vi "VR_WR.vi"(6 "Ydrp":dbl[](array[numeric]), 7 "Phirp":dbl[](array[numeric]), 9 "Xdrp":dbl[](array[numeric]), 10 "Phir":dbl[](array[numeric])) -> ()   [LabVIEW 2011]
uses:
  <vilib>/Analysis/Matrix/Datatypes/RealMatrix.ctl
  <vilib>/Analysis/Matrix/NI_Matrix.lvlib
panel:
  out "Real Matrix":T1
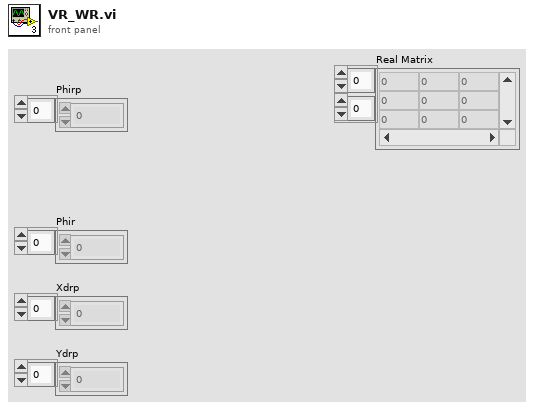
[diagram p1: front panel]
types:
  T1 = typedef "NI_Matrix.lvlib/RealMatrix.ctl" = dbl[][]
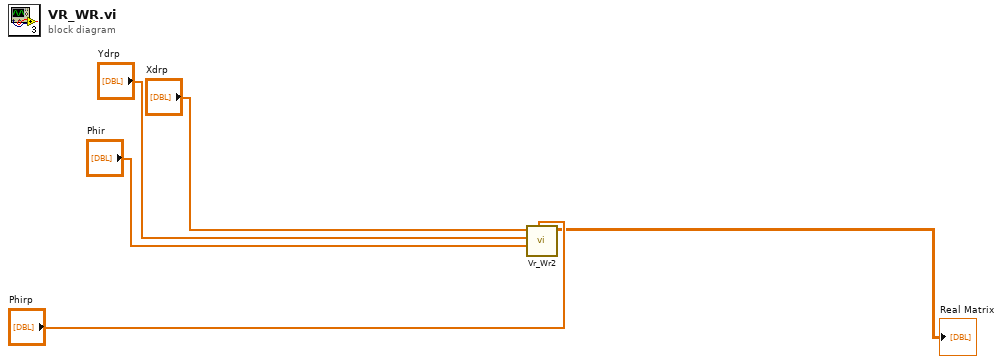
[diagram p0: block diagram]
diagram:
  n1 = call "Vr_Wr2.vi"("Phirp"="Phirp", "Phir"="Phir", "Ydrp"="Ydrp", "Xdrp"="Xdrp") -> ("VLW"=→"Real Matrix":T1)  [unwired: 7 in]
